vi "子VI-深度学习自动检测.vi"(8 "穿透图原始路径":path, 9 "产品规格":cluster{"产品长度（周长）（mm）":dbl, "产品宽度（母线长）（mm）":dbl}, 10 "临界面积百分比值":dbl, 11 "临界Z值":i32) -> (3 "全部检测结果":string[][](table))   [LabVIEW 2018]
panel:
  out "弥散类检测结果":string[][](table)
  in  "stop":bool caption="停止"
  out "模型预测进度（请等待2-3分钟）":u8(slide) scale=0.0..1000.0
  out "模型所在路径":path
  out "error out":errorcluster caption="错误输出"
  out "预测图片保存路径":path
  in  "选项卡控件":enum32{"原图", "预测结果", "分层类结果", "弥散类结果"}(tab)
  out "原图":T1(plugin-control)
  out "预测输出":T1(plugin-control)
  out "Threshold Image":T1(plugin-control)
  out "misan":T1(plugin-control)
  out "standard output":string
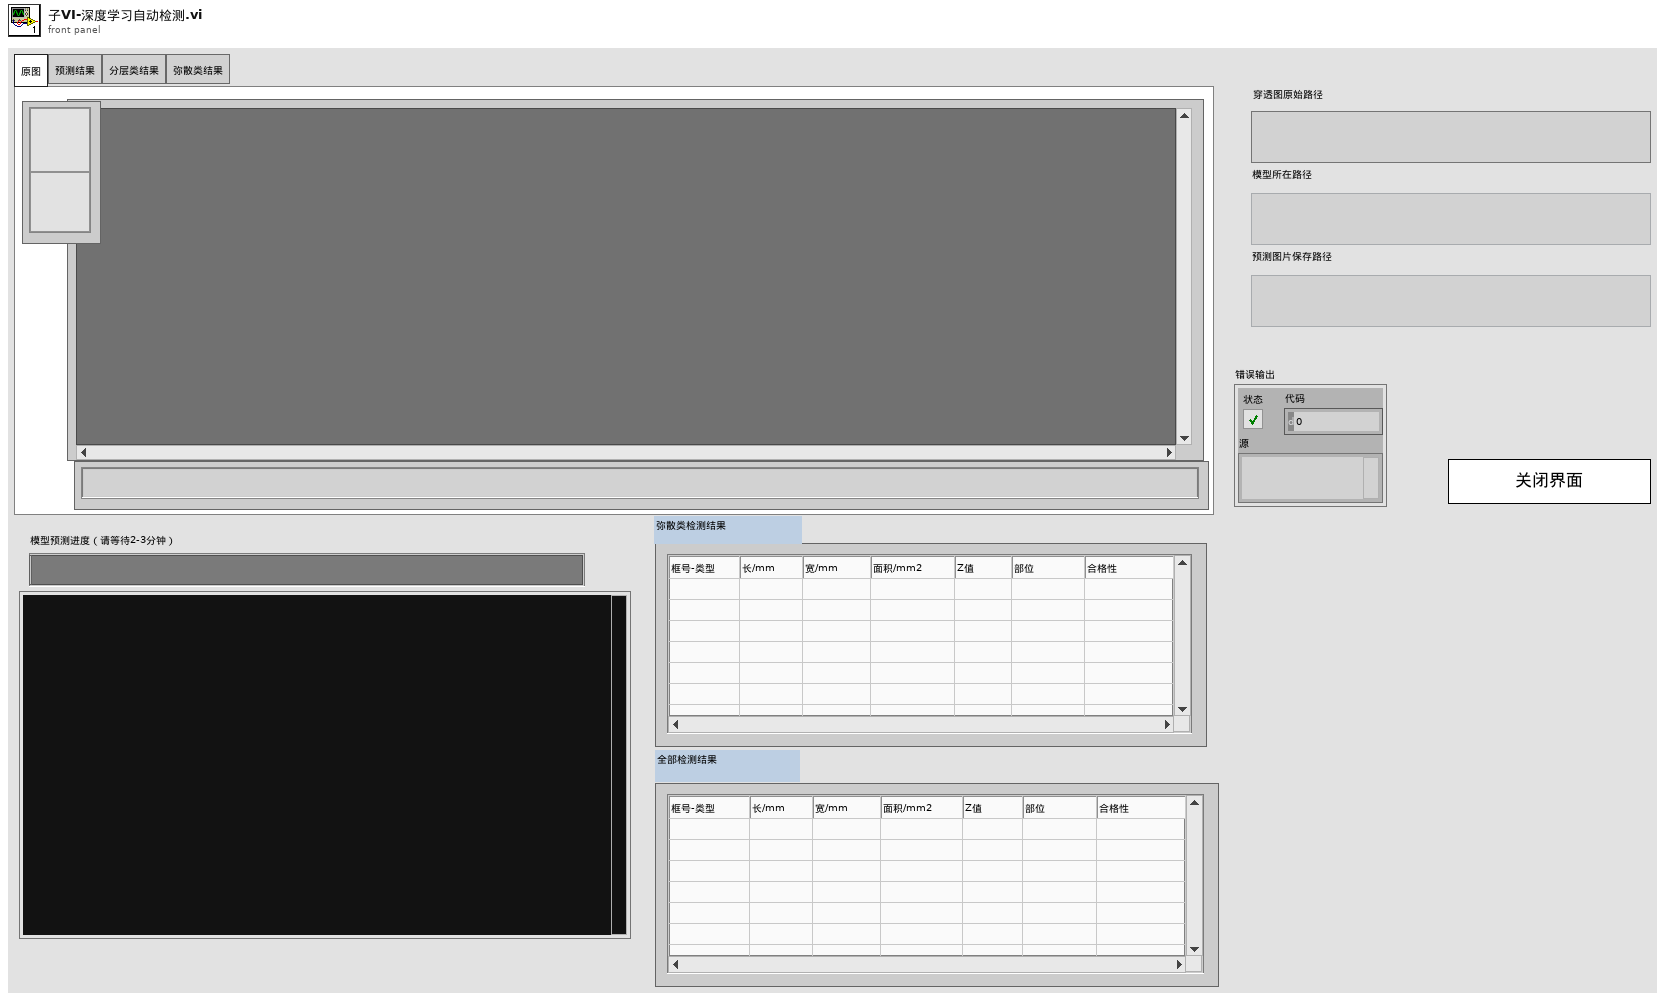
[diagram p1: front panel]
types:
  T1 = typedef "IMAQ Image.ctl" = refnum<image>
  T2 = typedef "Image Type" = u32
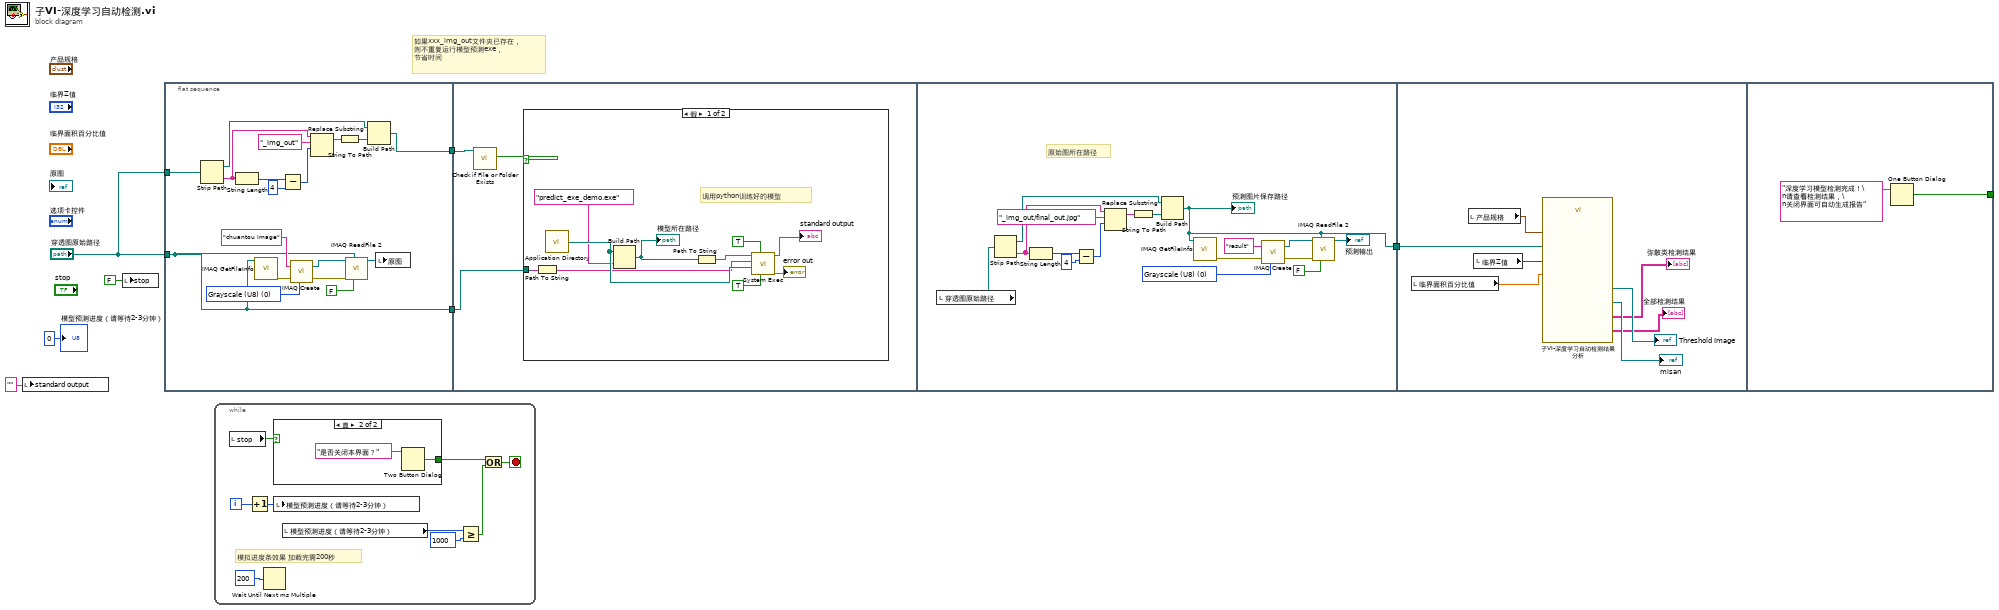
[diagram p0: block diagram]
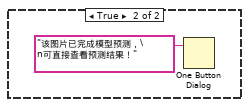
[diagram p2: hidden frame]
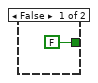
[diagram p3: hidden frame]
diagram:
  # "如果xxx_img_out文件夹已存在，\n则不重复运行模型预测exe，\n节省时间"
  n1 = local write "standard output"("" ("standard output")) -> ()
  n2 = local write "stop"(FALSE ("stop")) -> ()
  n3 = flat-sequence {
    tunnel: [w18] -> w5
    tunnel: "穿透图原始路径" -> [w18]
    tunnel: "穿透图原始路径" -> [w9]
    tunnel: [w8] -> w1
    tunnel: w5 -> [w27]
    tunnel: w1 -> [w28]
    tunnel: [w40] -> w4
    tunnel: w4 -> [w59]
    tunnel: [w65] -> _
    frame #0 {
      w20 = T2 0 items=["Grayscale (U8)", "Grayscale (I16)", "Grayscale (SGL)", "Complex (CSG)", "RGB (U32)", "HSL (U32)", "RGB (U64)", "Grayscale (U16)"] ("Image Type")
      n4 = Strip Path(path=w9) -> (stripped path=w16:path, name=w17:string)
      n5 = String Length(string=w17) -> (length=w14:i32)
      n6 = call "IMAQ GetFileInfo"("File Path"=w18) -> ("error out"=w23:errorcluster)  [unwired: 4 in, 6 out]
      n7 = Subtract(x=w14, y=4) -> (x-y=w13:i32)
      n8 = call "IMAQ Create"("Image Name"="chuantou Image", "Image Type"=w20, "error in (no error)"=w23) -> ("New Image"=w24:T1, "error out"=w25:errorcluster)  [unwired: 2 in]
      n9 = Replace Substring(3:w13, 4:"_img_out" ("字符串"), 5:w17) -> (1:w15:string)  [unwired: 1 in, 1 out]
      n10 = String To Path(string=w15) -> (path=w12:path)
      n11 = call "IMAQ ReadFile 2"("Use File Path Image Type"=FALSE, "File Path"=w18, "error in (no error)"=w25, "Image"=w24) -> ("Image Out"=w22:T1)  [unwired: 3 in, 4 out]
      n12 = Build Path(base path=w16, name or relative path=w12) -> (appended path=w8:path)
      n13 = local write "原图"(w22) -> ()
    }
    frame #1 {
      n14 = call <vilib>:"Check if File or Folder Exists.vi"("path"=w28) -> ("file or folder exists?"=w26:bool)  [unwired: 8 in, 2 out]
      n15 = case shown="假" w26 {
        tunnel: w27 -> [w29 _]
        frame False {
          # "调用python训练好的模型"
          n16 = Path To String(path=w29) -> (string=w35:string)
          n17 = call <vilib>:"Application Directory.vi"() -> ("Application Directory"=w36:path)
          n18 = Build Path(base path=w36, name or relative path="predict_exe_demo.exe" ("名称或相对路径")) -> (appended path=w37:path)
          "模型所在路径" <- w37
          n19 = Path To String(path=w37) -> (string=w38:string)
          n20 = call <vilib>:"System Exec.vi"("run minimized? (F)"=TRUE, "wait until completion? (T)"=TRUE, "working directory"=w36, "standard input"=w35, "command line"=w38) -> ("error out"=→"error out":errorcluster, "standard output"=→"standard output":string)  [unwired: 3 in, 2 out]
        }
        frame True {
          n21 = One Button Dialog(message="该图片已完成模型预测，\n可直接查看预测结果！" ("消息")) -> ()  [unwired: 1 in, 1 out]
        }
      }
    }
    frame #2 {
      w52 = T2 0 items=["Grayscale (U8)", "Grayscale (I16)", "Grayscale (SGL)", "Complex (CSG)", "RGB (U32)", "HSL (U32)", "RGB (U64)", "Grayscale (U16)"] ("Image Type")
      # "原始图所在路径"
      n22 = local read "穿透图原始路径"() -> (w41:path)
      n23 = Strip Path(path=w41) -> (stripped path=w43:path, name=w42:string)
      n24 = String Length(string=w42) -> (length=w47:i32)
      n25 = Subtract(x=w47, y=4) -> (x-y=w48:i32)
      n26 = Replace Substring(3:w48, 4:"_img_out/final_out.jpg" ("字符串"), 5:w42) -> (1:w46:string)  [unwired: 1 in, 1 out]
      n27 = String To Path(string=w46) -> (path=w49:path)
      n28 = Build Path(base path=w43, name or relative path=w49) -> (appended path=w40:path)
      "预测图片保存路径" <- w40
      n29 = call "IMAQ GetFileInfo"("File Path"=w40) -> ("error out"=w54:errorcluster)  [unwired: 4 in, 6 out]
      n30 = call "IMAQ Create"("Image Name"="result", "Image Type"=w52, "error in (no error)"=w54) -> ("New Image"=w55:T1, "error out"=w56:errorcluster)  [unwired: 2 in]
      n31 = call "IMAQ ReadFile 2"("Use File Path Image Type"=FALSE, "File Path"=w40, "error in (no error)"=w56, "Image"=w55) -> ("Image Out"=→"预测输出":T1)  [unwired: 3 in, 4 out]
    }
    frame #3 {
      n32 = local read "临界面积百分比值"() -> (w62:dbl)
      n33 = local read "产品规格"() -> (w64:cluster{"产品长度（周长）（mm）":dbl, "产品宽度（母线长）（mm）":dbl})
      n34 = local read "临界Z值"() -> (w63:i32)
      n35 = call "子VI-深度学习自动检测结果分析.vi"("临界Z值"=w63, "临界面积百分比值"=w62, "预测图片保存路径"=w59, "产品规格"=w64) -> ("全部检测结果"=→"全部检测结果":string[][], "弥散类检测结果"=→"弥散类检测结果":string[][], 17:→"Threshold Image":T1, 18:→"misan":T1)  [unwired: 12 in]
    }
    frame #4 {
      n36 = One Button Dialog(message="深度学习模型检测完成！\n请查看检测结果，\n关闭界面可自动生成报告" ("消息")) -> (true=w65:bool)  [unwired: 1 in]
    }
  }
  n37 = while {
    i -> [w68]
    stop <- w71 stop-if-true
    # "模拟进度条效果 加载完需200秒"
    n38 = local read "stop"() -> (w70:bool)
    n39 = Increment(x=w68) -> (x+1=w67:i32)
    n40 = Wait Until Next ms Multiple(millisecond multiple=u32 200 ("毫秒倍数")) -> ()  [unwired: 1 out]
    n41 = case shown="真" w70 {
      tunnel: [FALSE ("T button?") w77] -> w69
      frame False {
      }
      frame True {
        n42 = Two Button Dialog(message="是否关闭本界面？" ("消息")) -> (T button?=w77:bool)  [unwired: 2 in]
      }
    }
    n43 = local write "模型预测进度（请等待2-3分钟）"(w67) -> ()
    n44 = local read "模型预测进度（请等待2-3分钟）"() -> (w73:u8)
    n45 = Greater Or Equal?(x=w73, y=1000) -> (x >= y?=w72:bool)
    n46 = Or(x=w69, y=w72) -> (x .or. y?=w71:bool)
  }
  "模型预测进度（请等待2-3分钟）" <- u8 0 ("模型运行进度")
